vi "BallReplacement Packet Encoder.vi"(11 "grSim_BallReplacement":T1) -> (1 "Array":u8[](array[numeric]))   [LabVIEW 2018]
uses:
  grSim_BallReplacement.ctl
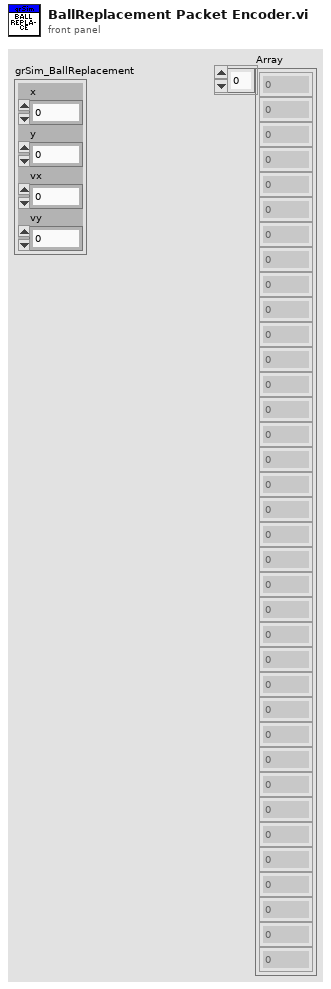
[diagram p1: front panel]
types:
  T1 = typedef "grSim_BallReplacement.ctl" = cluster{"x":dbl, "y":dbl, "vx":dbl, "vy":dbl}
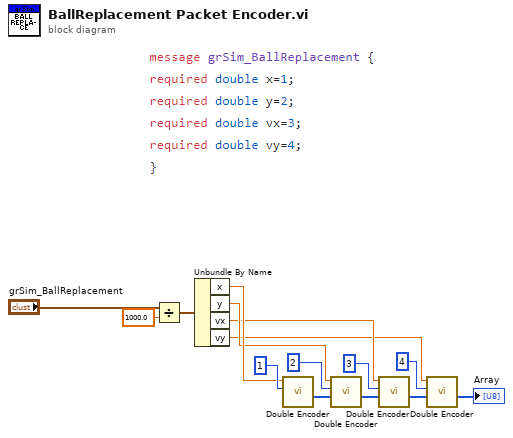
[diagram p0: block diagram]
diagram:
  n1 = Divide(x="grSim_BallReplacement", y=1000.0) -> (x/y=w1:T1)
  n2 = Unbundle By Name(w1) -> ("x"=w7:dbl, "y"=w6:dbl, "vx"=w5:dbl, "vy"=w4:dbl)
  n3 = call "Double Encoder.vi"("Key"=u32 1, "Value"=w7) -> ("Array"=w13:u8[])  [unwired: 9 in]
  n4 = call "Double Encoder.vi"("Array In"=w13, "Key"=u32 2, "Value"=w6) -> ("Array"=w12:u8[])  [unwired: 8 in]
  n5 = call "Double Encoder.vi"("Array In"=w12, "Key"=u32 3, "Value"=w5) -> ("Array"=w11:u8[])  [unwired: 8 in]
  n6 = call "Double Encoder.vi"("Array In"=w11, "Key"=u32 4, "Value"=w4) -> ("Array"=→"Array":u8[])  [unwired: 8 in]
